vi "Get as LabVIEW type (poly).vi"   [LabVIEW 2020, in "JSONtext.lvlib"]
doc: "Convert a JSON Value into a LabVIEW data type. Polymorphic; select the type of data. Type may also be specified by a supplied type in a Variant. This may be a cluster of other types."
uses:
  <vilib>/JDP Science/JSONtext/JSONtext.lvlib
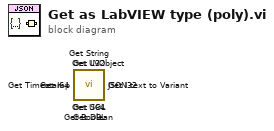
[diagram p0: block diagram]
diagram:
  n1 = call <vilib>:"Get SGL.vi"() -> ()  [unwired: 9 in, 3 out]
  n2 = call <vilib>:"Get LVObject.vi"() -> ()  [unwired: 9 in, 3 out]
  n3 = call <vilib>:"Get Timestamp.vi"() -> ()  [unwired: 9 in, 3 out]
  n4 = call <vilib>:"JSON text to Variant.vi"() -> ()  [unwired: 10 in, 2 out]
  n5 = call <vilib>:"Get Boolean.vi"() -> ()  [unwired: 9 in, 3 out]
  n6 = call <vilib>:"Get String.vi"() -> ()  [unwired: 9 in, 3 out]
  n7 = call <vilib>:"Get U64.vi"() -> ()  [unwired: 9 in, 3 out]
  n8 = call <vilib>:"Get U32.vi"() -> ()  [unwired: 9 in, 3 out]
  n9 = call <vilib>:"Get I64.vi"() -> ()  [unwired: 9 in, 3 out]
  n10 = call <vilib>:"Get I32.vi"() -> ()  [unwired: 9 in, 3 out]
  n11 = call <vilib>:"Get DBL.vi"() -> ()  [unwired: 9 in, 3 out]
